vi "LUnit CLI Post-Install.vi"(9 "operations directory override":string, 10 "source directory override":string, 11 "Variant":variant) -> (0 "error out":errorcluster, 3 "operation path":path)   [LabVIEW 2020]
doc: "VIPM post-install custom action for LUnit CLI.\n\nCopies the LUnitCLI operation folder from vi.lib/Astemes/LUnit CLI/LUnitCLI into the LabVIEW CLI Operations directory so that LabVIEWCLI -OperationName LUnit finds it. The Operations directory is the first of these that exists (checked at run time because LabVIEW before 2025 does not evaluate the OS conditional symbol reliably outside a project):\n Windows: C:/Program Files (x86)/National Instruments/Shared/LabVIEW CLI/Operations\n Linux: /usr/local/natinst/nilvcli/Operations\n macOS: /Library/Application Support/National Instruments/LabVIEW CLI/Operations\nAn existing LUnitCLI folder there is replaced. Writing there needs administrator (Windows) or root (Linux/macOS) rights. If the copy fails error out explains how to use -AdditionalOperationDirectory instead.\n\nThe two override inputs exist for testing only. VIPM leaves them empty."
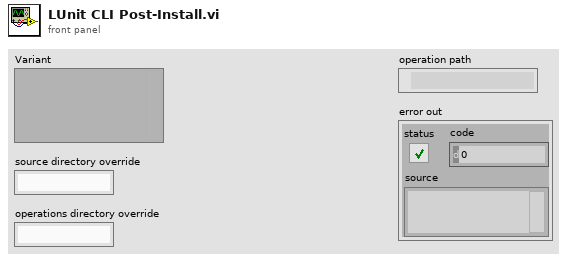
[diagram p1: front panel]
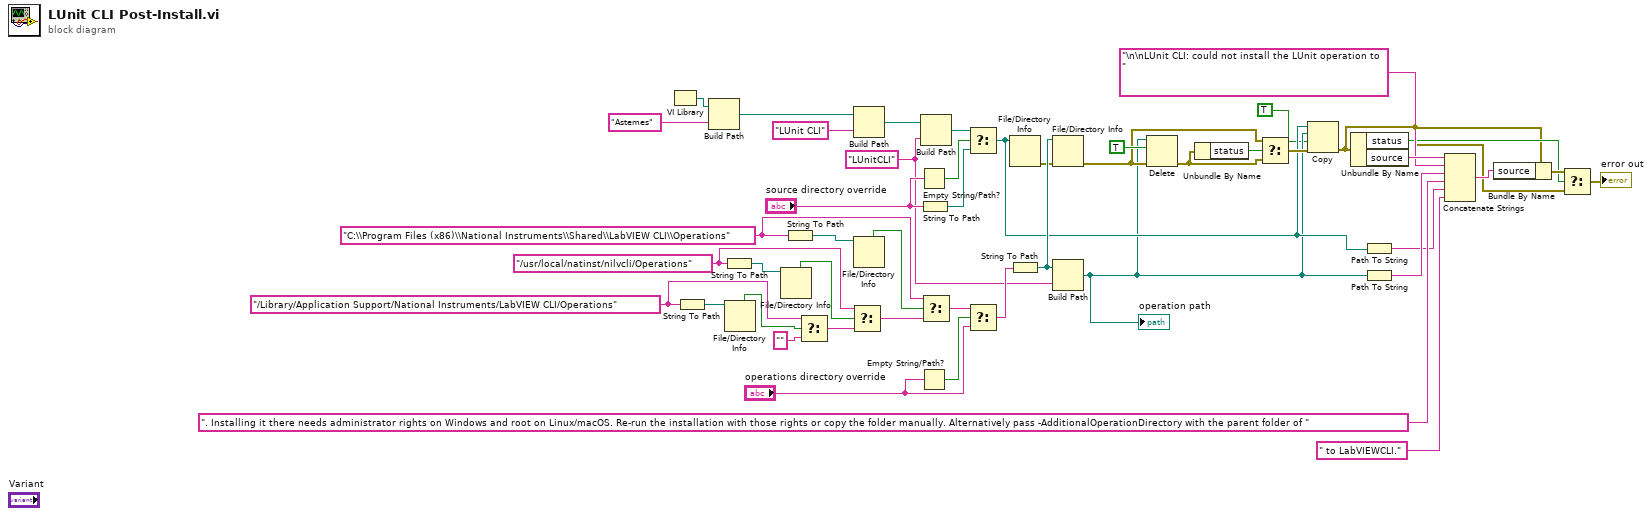
[diagram p0: block diagram]
diagram:
  w35 = "/Library/Application Support/National Instruments/LabVIEW CLI/Operations"
  w32 = "/usr/local/natinst/nilvcli/Operations"
  w29 = "C:\\Program Files (x86)\\National Instruments\\Shared\\LabVIEW CLI\\Operations"
  w22 = "LUnitCLI"
  n1 = VI Library() -> (path=w47:path)
  n2 = String To Path(string=w35) -> (path=w36:path)
  n3 = Build Path(base path=w47, name or relative path="Astemes") -> (appended path=w45:path)
  n4 = String To Path(string=w32) -> (path=w37:path)
  n5 = File/Directory Info(path=w36) -> (directory=w34:bool)  [unwired: 1 in, 6 out]
  n6 = File/Directory Info(path=w37) -> (directory=w31:bool)  [unwired: 1 in, 6 out]
  n7 = String To Path(string=w29) -> (path=w38:path)
  n8 = Select(t=w35, s=w34, f="") -> (s? t:f=w30:string)
  n9 = Select(t=w32, s=w31, f=w30) -> (s? t:f=w27:string)
  n10 = Build Path(base path=w45, name or relative path="LUnit CLI") -> (appended path=w43:path)
  n11 = File/Directory Info(path=w38) -> (directory=w28:bool)  [unwired: 1 in, 6 out]
  n12 = Empty String/Path?(string/path="source directory override") -> (empty?=w40:bool)
  n13 = Empty String/Path?(string/path="operations directory override") -> (empty?=w25:bool)
  n14 = String To Path(string="source directory override") -> (path=w39:path)
  n15 = Build Path(base path=w43, name or relative path=w22) -> (appended path=w41:path)
  n16 = Select(t=w29, s=w28, f=w27) -> (s? t:f=w26:string)
  n17 = Select(t=w41, s=w40, f=w39) -> (s? t:f=w14:path)
  n18 = Select(t=w26, s=w25, f="operations directory override") -> (s? t:f=w23:string)
  n19 = File/Directory Info(path=w14) -> (error out=w20:errorcluster)  [unwired: 1 in, 6 out]
  n20 = String To Path(string=w23) -> (path=w21:path)
  n21 = File/Directory Info(path=w21, error in=w20) -> (error out=w18:errorcluster)  [unwired: 6 out]
  n22 = Build Path(base path=w21, name or relative path=w22) -> (appended path=w3:path)
  "operation path" <- w3
  n23 = Delete(path (use dialog)=w3, entire hierarchy (F)=TRUE, error in=w18) -> (error out=w16:errorcluster)  [unwired: 2 in, 2 out]
  n24 = Unbundle By Name(w16) -> ("status"=w17:bool)
  n25 = Select(t=w18, s=w17, f=w16) -> (s? t:f=w15:errorcluster)
  n26 = Copy(8:w15, 9:TRUE ("overwrite (F)"), 10:w3, 11:w14) -> (0:w4:errorcluster)  [unwired: 1 in, 2 out]
  n27 = Unbundle By Name(w4) -> ("status"=w5:bool, "source"=w13:string)
  n28 = Path To String(path=w14) -> (string=w9:string)
  n29 = Path To String(path=w3) -> (string=w11:string)
  n30 = Concatenate Strings(w13, "\n\nLUnit CLI: could not install the LUnit operation to ", w11, ". Installing it there needs administrator rights on Windows and root on Linux/macOS. Re-run the installation with those rights or copy the folder manually. Alternatively pass -AdditionalOperationDirectory with the parent folder of ", w9, " to LabVIEWCLI.") -> (w7:string)
  n31 = Bundle By Name(cluster=w4, "source"=w7) -> (w6:errorcluster)
  n32 = Select(t=w6, s=w5, f=w4) -> (s? t:f=→"error out":errorcluster)
